vi "LCA Set Default Pos Unit.vi"(7 "Prefix":T2=-3 items=["UNIT"=0, "DECI"=-1, "CENTI"=-2, "MILLI"=-3, "MICRO"=-6], 8 "error in (no error)":errorcluster caption="Fehler (Eingang, kein Fehler)", 10 "Position Unit":T1 items=["METERS", "REVOLUTIONS", "DEGREE", "RADIAN", "DEVICE"], 11 "Axis Handle":i64) -> (0 "error out":errorcluster caption="Fehler (Ausgang)")   [LabVIEW 2021, in "labbCAN_MotionControl_API.lvlib"]
doc: "LCA_Func long __stdcall LCA_SetDefaultPosUnit(dev_hdl hAxis,\n char Prefix,\n int PositionUnit);"
uses:
  labbCAN_MotionControl_API.lvlib
  labbCAN_Bus_API/SiUnitPrefix.ctl
  PositionUnits.ctl
  labbCAN_MotionControl_API.dll
  labbCAN_Bus_API/labbCAN_Bus_API.lvlib
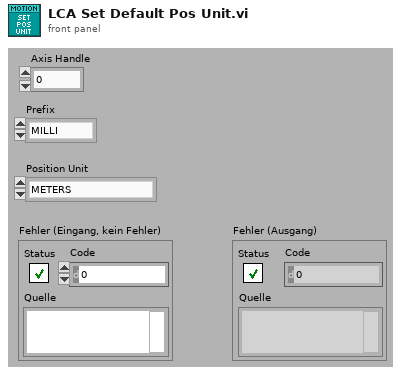
[diagram p1: front panel]
types:
  T1 = typedef "labbCAN_MotionControl_API.lvlib/PositionUnits.ctl" = i32
  T2 = typedef "labbCAN_Bus_API.lvlib/SiUnitPrefix.ctl" = i32
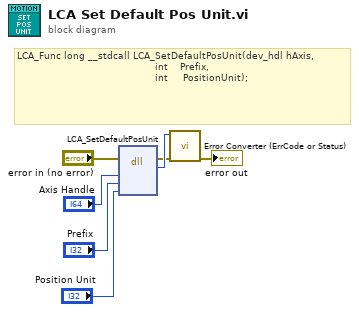
[diagram p0: block diagram]
diagram:
  # "LCA_Func long __stdcall LCA_SetDefaultPosUnit(dev_hdl hAxis,\n                                              int    Prefix,\n                                              int     PositionUnit);"
  n1 = dll-call lib="C:/Users/olaja/AppData/Local/CETONI_SDK/labbCAN_MotionControl_API.*" fn="LCA_SetDefaultPosUnit"(error in="error in (no error)", "hAxis"="Axis Handle", "Prefix"="Prefix", "PositionUnit"="Position Unit") -> (error out=w2:errorcluster, "Rückgabetyp"=w7:i32)  [unwired: 5 in, 1 out]
  n2 = call "Error Converter (ErrCode or Status).vi"("error in (no error)"=w2, "error code"=w7) -> ("error out"=→"error out":errorcluster)  [unwired: 9 in]
